vi "write_pico_file_binary.vi"(8 "Pico Data In":dbl[][](array[numeric]), 9 "Raw Data Folder":path, 10 "Filename":string, 11 "Use Channel":bool) -> ()   [LabVIEW 2016]
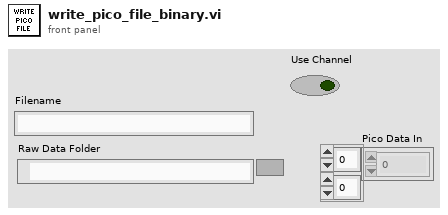
[diagram p1: front panel]
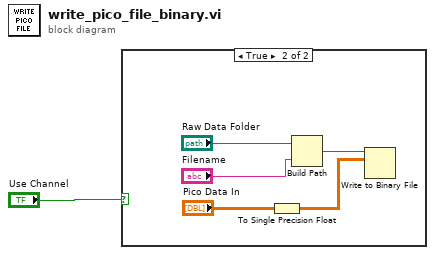
[diagram p0: block diagram]
diagram:
  n1 = case shown="True" "Use Channel" {
    frame False {
    }
    frame True {
      n2 = To Single Precision Float(number="Pico Data In") -> (single precision float=w2:sgl[][])
      n3 = Build Path(base path="Raw Data Folder", name or relative path="Filename") -> (appended path=w5:path)
      n4 = Write to Binary File(file (use dialog)=w5, data=w2) -> ()  [unwired: 4 in, 3 out]
    }
  }
